vi "readDataArray.vi"(8 "error in (no error)":errorcluster, 10 "array":string[][](array[string]), 11 "FileReader in":refnum<class "FileReader.lvclass">) -> (0 "error out":errorcluster, 3 "FileReader out":refnum<class "FileReader.lvclass">)   [LabVIEW 2011, in "Tools.lvlib" / "Filing.lvlib" / "FileReader.lvclass"]
uses:
  FileReader.lvclass
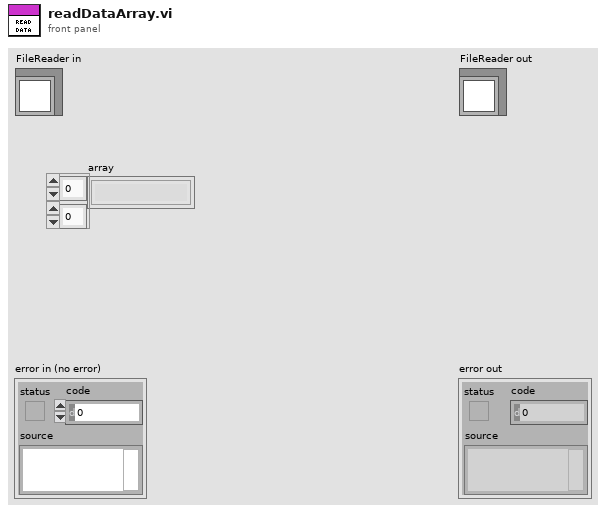
[diagram p1: front panel]
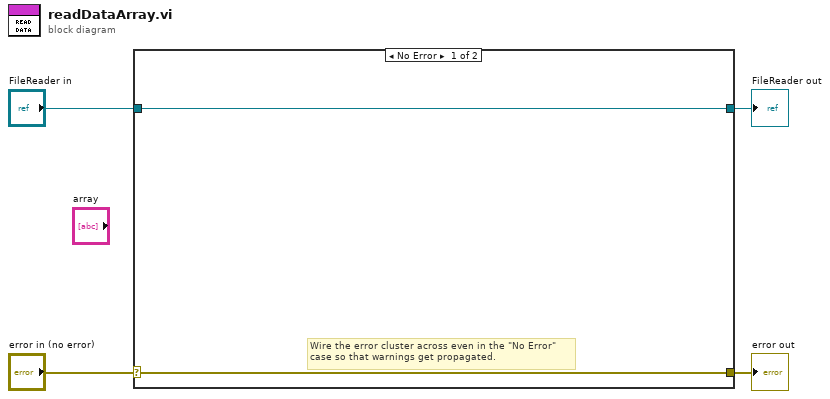
[diagram p0: block diagram]
diagram:
  n1 = case shown="No Error" "error in (no error)" {
    selector: "error in (no error)" -> [w5 w8]
    tunnel: [w5 w8] -> w3
    tunnel: [w6 w7] -> w1
    tunnel: "FileReader in" -> [w6 w7]
    frame No Error {
      # "Wire the error cluster across even in the \"No Error\"\ncase so that warnings get propagated."
    }
    frame Error {
    }
  }
  "error out" <- w3
  "FileReader out" <- w1
